vi "Esercitazione 1 - Equal led on.vi"() -> ()   [LabVIEW 2018]
panel:
  out "Led":bool
  in  "Operatore 2":i32(knob) scale=0.0..10.0
  in  "Operatore 1":i32(knob) scale=0.0..10.0
  # "equal led on=\naccendi led quando due num int ingresso sono uguali"
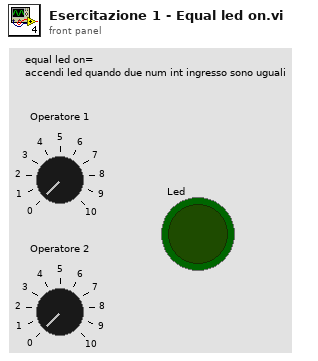
[diagram p1: front panel]
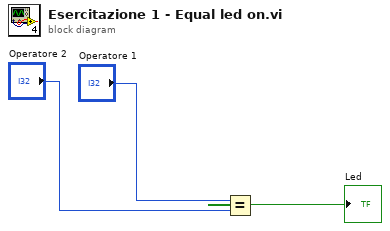
[diagram p0: block diagram]
diagram:
  n1 = Equal?(x="Operatore 1", y="Operatore 2") -> (x = y?=→"Led":bool)
